vi "sysm excu.vi"() -> ()   [LabVIEW 2011]
panel:
  out "standard output 3":string
  in  "standard input":string
  in  "command line":string
  out "standard output 2":string
  out "standard output":string
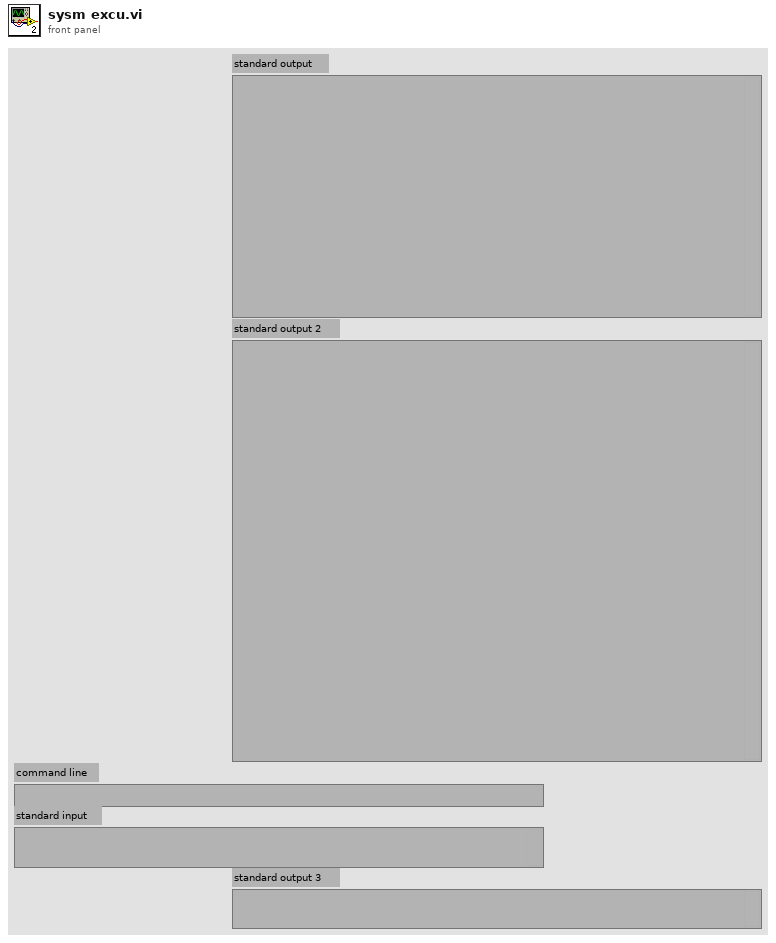
[diagram p1: front panel]
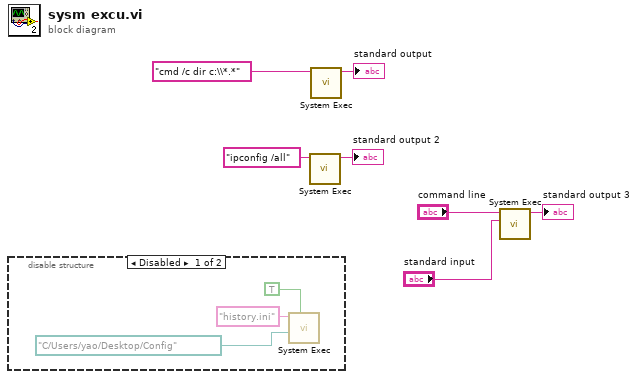
[diagram p0: block diagram]
diagram:
  n1 = disable-structure shown="Disabled" {
    frame Disabled {
      n2 = call <vilib>:"System Exec.vi"("wait until completion? (T)"=TRUE, "working directory"=path "C:/Users/yao/Desktop/Config", "command line"="history.ini") -> ()  [unwired: 5 in, 4 out]
    }
    frame Enabled {
    }
  }
  n3 = call <vilib>:"System Exec.vi"("command line"="ipconfig /all") -> ("standard output"=→"standard output 2":string)  [unwired: 7 in, 3 out]
  n4 = call <vilib>:"System Exec.vi"("command line"="cmd /c dir c:\\*.*") -> ("standard output"=→"standard output":string)  [unwired: 7 in, 3 out]
  n5 = call <vilib>:"System Exec.vi"("standard input"="standard input", "command line"="command line") -> ("standard output"=→"standard output 3":string)  [unwired: 6 in, 3 out]
